vi "Balansing logic.vi"(9 "Vmax":dbl, 10 "Vmin":dbl, 11 "Voltage":dbl[](array[numeric])) -> (2 "error constant":errorcluster, 3 "Array":bool[](array[boolean]))   [LabVIEW 2026]
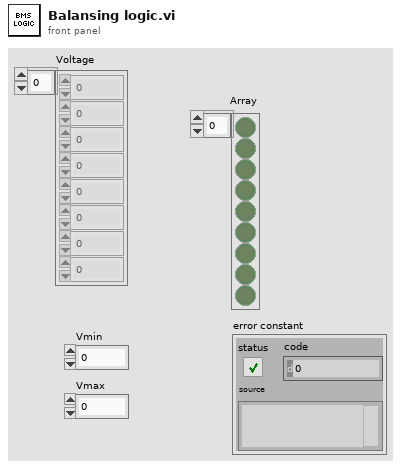
[diagram p1: front panel]
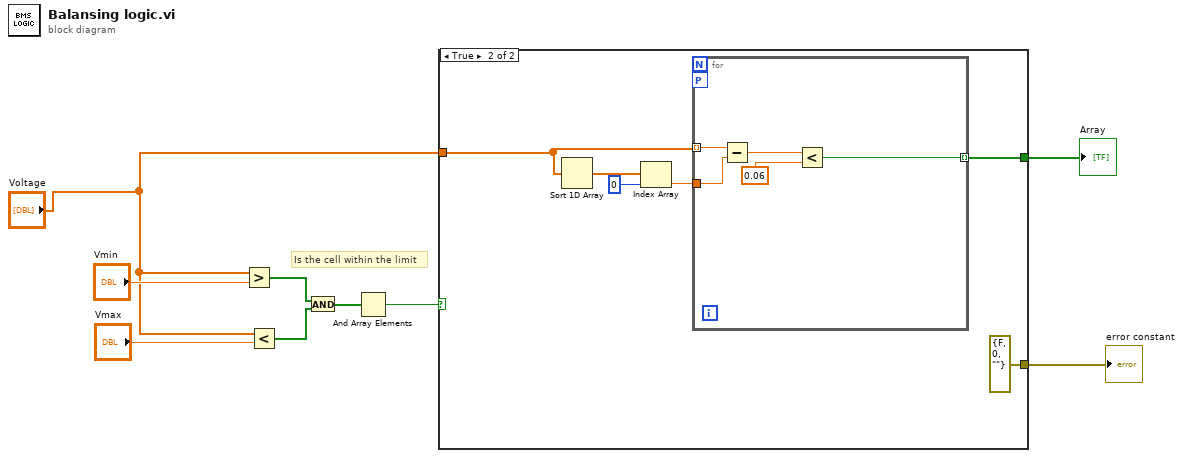
[diagram p0: block diagram]
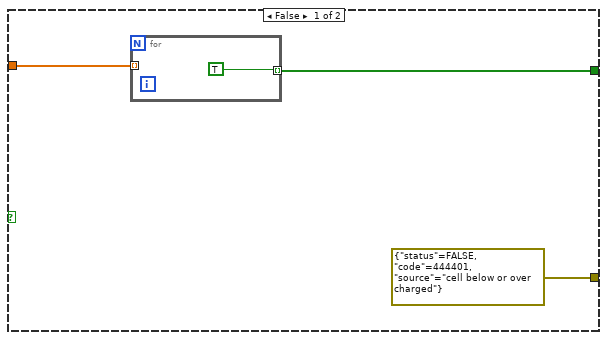
[diagram p2: hidden frame]
diagram:
  # "Is the cell within the limit"
  n1 = Greater?(x="Voltage", y="Vmin") -> (0:w7:bool[])
  n2 = Less?(x="Voltage", y="Vmax") -> (x < y?=w6:bool[])
  n3 = And(x=w7, y=w6) -> (x .and. y?=w5:bool[])
  n4 = And Array Elements(Boolean array=w5) -> (logical AND=w4:bool)
  n5 = case shown="True" w4 {
    tunnel: [errorcluster {"status"=FALSE, "code"=444401, "source"="cell below or over charged"} ("error constant") errorcluster {"status"=FALSE, "code"=0, "source"=""} ("error constant")] -> w2
    tunnel: "Voltage" -> [w11 w16]
    tunnel: [w10 w14] -> w3
    frame False {
      n6 = for {
        tunnel: w11 -> [_] mode=indexing
        tunnel: [TRUE] -> w10 mode=indexing
      }
    }
    frame True {
      n7 = Sort 1D Array(array=w16) -> (sorted array=w19:dbl[])
      n8 = Index Array(array=w19, index=0) -> (element=w17:dbl)
      n9 = for {
        tunnel: w17 -> [w24]
        tunnel: w16 -> [w23] mode=indexing
        workers-P: _ -> [_]
        tunnel: [w20] -> w14 mode=indexing
        n10 = Subtract(x=w23, y=w24) -> (x-y=w22:dbl)
        n11 = Less?(x=w22, y=0.06) -> (x < y?=w20:bool)
      }
    }
  }
  "Array" <- w3
  "error constant" <- w2
